vi "python_node_example_2023_Q3.vi"() -> ()   [LabVIEW 2021]
panel:
  out "return_tuple":cluster{i32, i32, bool[]}
  out "return_dict":T1
  out "return_tuple_list":cluster{i32, i32, bool[]}[](array[cluster])
  out "return_list":bool[](array[boolean])
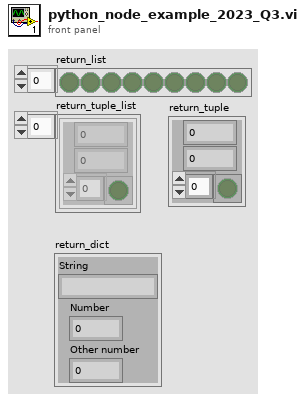
[diagram p1: front panel]
types:
  T1 = cluster{"String":string, "Number":i32, "Other number":i32}
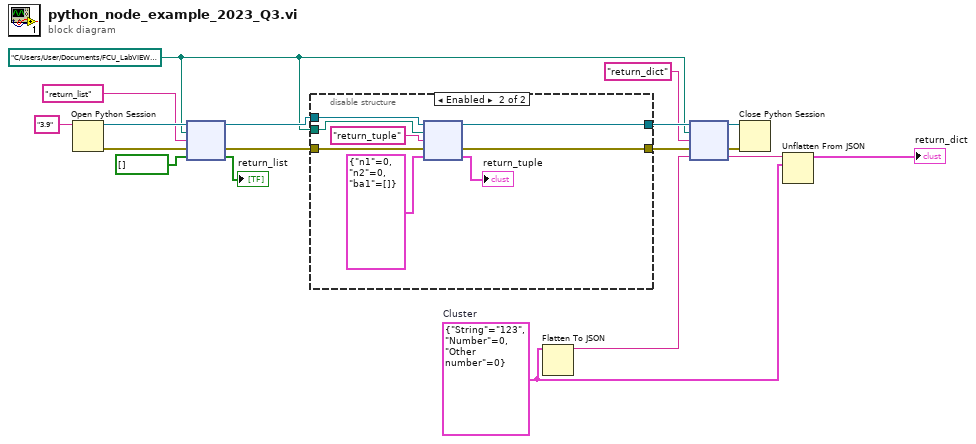
[diagram p0: block diagram]
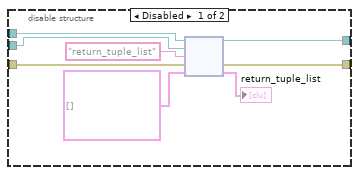
[diagram p2: hidden frame]
diagram:
  w4 = T1 {"String"="123", "Number"=0, "Other number"=0}  # Cluster
  w2 = path "C:/Users/User/Documents/FCU_LabVIEW_Course_AI_part/python_node_example.py" ("module path")
  n1 = Open Python Session(python version="3.9" ("Python version")) -> (session out=w18:refnum<k35>, error out=w17:errorcluster)  [unwired: 2 in]
  n2 = node(w18, w2, "return_list" ("function name"), w17, bool[] []) -> (w12:refnum<k35>, w11:errorcluster, →"return_list":bool[])  [unwired: 2 out]
  n3 = disable-structure shown="Enabled" {
    disable-tunnel: w12 -> [w25 w33]
    disable-tunnel: w11 -> [w24 w32]
    disable-tunnel: [w23 w31] -> w10
    disable-tunnel: [w22 w30] -> w9
    disable-tunnel: w2 -> [w19 w29]
    frame Disabled {
      n4 = node(w25, w19, "return_tuple_list" ("function name"), w24, cluster{i32, i32, bool[]}[] []) -> (w23:refnum<k35>, w22:errorcluster, →"return_tuple_list":cluster{i32, i32, bool[]}[])  [unwired: 2 out]
    }
    frame Enabled {
      n5 = node(w33, w29, "return_tuple" ("function name"), w32, cluster{"n1":i32, "n2":i32, "ba1":bool[]} {"n1"=0, "n2"=0, "ba1"=[]} ("Cluster")) -> (w31:refnum<k35>, w30:errorcluster, →"return_tuple":cluster{"n1":i32, "n2":i32, "ba1":bool[]})  [unwired: 2 out]
    }
  }
  n6 = Flatten To JSON(anything=w4) -> (JSON string=w6:string)  [unwired: 2 in, 1 out]
  n7 = node(w10, w2, "return_dict" ("function name"), w9, w6) -> (w14:refnum<k35>, w13:errorcluster, w5:string)  [unwired: 2 out]
  n8 = Close Python Session(session in=w14, error in=w13) -> ()  [unwired: 1 out]
  n9 = Unflatten From JSON(JSON string=w5, type and defaults=w4) -> (value=→"return_dict":T1)  [unwired: 5 in, 1 out]
